vi "kreator_siatki.vi"(2 "error in (no error)":errorcluster, 3 "Liczba Przejść":i32, 4 "Wektor 2":dbl[](array[numeric]), 5 "Wektor 1":dbl[](array[numeric])) -> (0 "error out":errorcluster, 1 "Tablica pkt":dbl[][][](array[numeric]))   [LabVIEW 2016]
doc: "To subvi zwraca tablice pkt. stworzonych z przyjętych wektorów bazowych , oddalonych od zera od zadanej liczbie przejść"
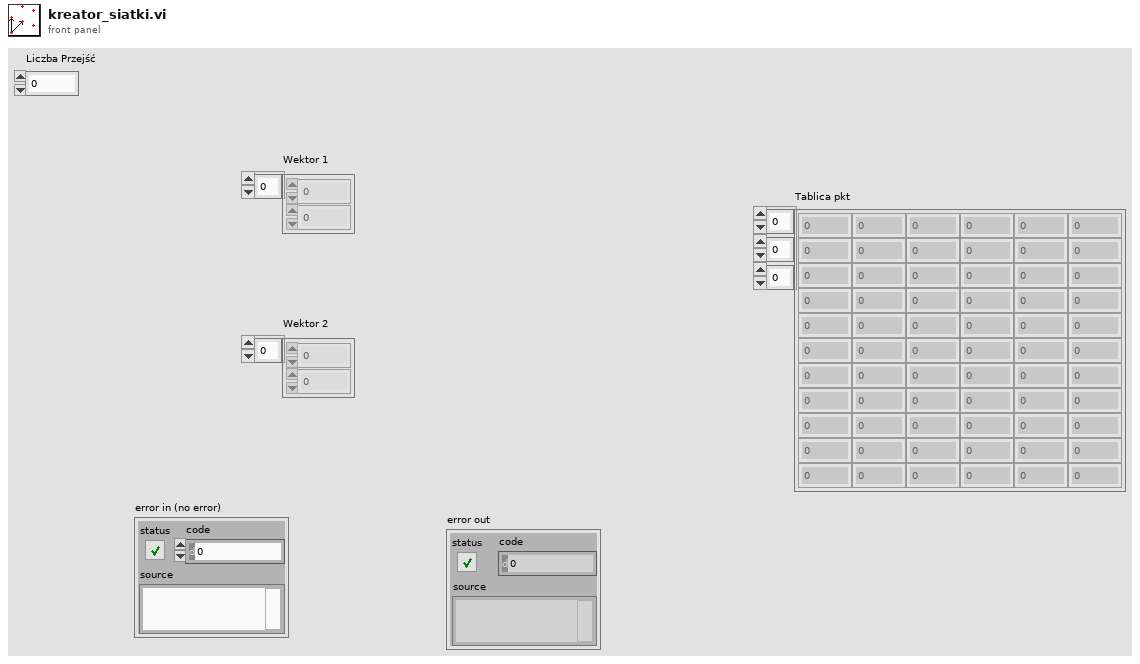
[diagram p1: front panel]
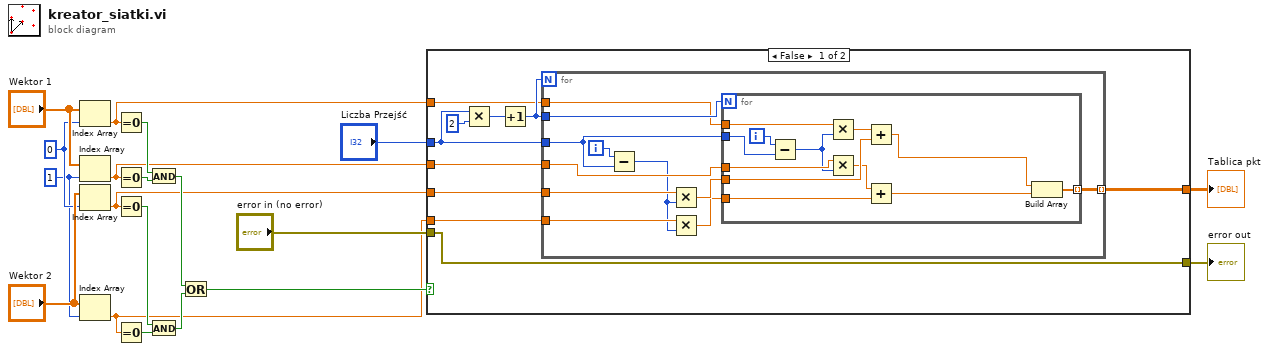
[diagram p0: block diagram]
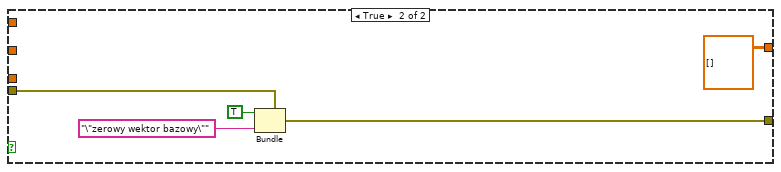
[diagram p2: hidden frame]
diagram:
  w16 = 1 ("index")
  w17 = 0 ("index")
  n1 = Index Array(array="Wektor 1", index=w17) -> (element=w5:dbl)
  n2 = Index Array(array="Wektor 1", index=w16) -> (element=w4:dbl)
  n3 = Index Array(array="Wektor 2", index=w17) -> (element=w3:dbl)
  n4 = Index Array(array="Wektor 2", index=w16) -> (element=w2:dbl)
  n5 = Equal To 0?(x=w5) -> (x = 0?=w15:bool)
  n6 = Equal To 0?(x=w4) -> (x = 0?=w14:bool)
  n7 = Equal To 0?(x=w3) -> (x = 0?=w13:bool)
  n8 = Equal To 0?(x=w2) -> (x = 0?=w12:bool)
  n9 = And(x=w15, y=w14) -> (x .and. y?=w11:bool)
  n10 = And(x=w13, y=w12) -> (x .and. y?=w10:bool)
  n11 = Or(x=w11, y=w10) -> (x .or. y?=w9:bool)
  n12 = case shown="False" w9 {
    tunnel: "error in (no error)" -> [w29 w57]
    tunnel: [w29 w54] -> w7
    tunnel: "Liczba Przejść" -> [w20 _]
    tunnel: w5 -> [w27 _]
    tunnel: w4 -> [w26 _]
    tunnel: w3 -> [w25 _]
    tunnel: w2 -> [w24 _]
    tunnel: [w23 dbl[][][] []] -> w1
    frame False {
      n13 = Multiply(x=w20, y=2) -> (x*y=w21:i32)
      n14 = Increment(x=w21) -> (x+1=w28:i32)
      n15 = for {
        N: w28 -> [_]
        tunnel: w28 -> [w40]
        tunnel: w27 -> [w39]
        tunnel: w26 -> [w38]
        tunnel: w25 -> [w37]
        tunnel: w24 -> [w36]
        tunnel: [w33] -> w23 mode=indexing
        tunnel: w20 -> [w32]
        i -> [w31]
        n16 = Subtract(x=w31, y=w32) -> (x-y=w30:i32)
        n17 = Multiply(x=w37, y=w30) -> (x*y=w35:dbl)
        n18 = Multiply(x=w36, y=w30) -> (x*y=w34:dbl)
        n19 = for {
          N: w40 -> [_]
          tunnel: w39 -> [w52]
          tunnel: w38 -> [w51]
          tunnel: w35 -> [w49]
          tunnel: w34 -> [w48]
          tunnel: [w44] -> w33 mode=indexing
          tunnel: w32 -> [w43]
          i -> [w42]
          n20 = Subtract(x=w42, y=w43) -> (x-y=w41:i32)
          n21 = Multiply(x=w52, y=w41) -> (x*y=w50:dbl)
          n22 = Multiply(x=w51, y=w41) -> (x*y=w47:dbl)
          n23 = Add(x=w50, y=w49) -> (x+y=w46:dbl)
          n24 = Add(x=w47, y=w48) -> (x+y=w45:dbl)
          n25 = Build Array(w46, w45) -> (w44:dbl[])
        }
      }
    }
    frame True {
      n26 = Bundle(cluster=w57, "status"=TRUE, "source"="\"zerowy wektor bazowy\"") -> (w54:errorcluster)  [unwired: 1 in]
    }
  }
  "error out" <- w7
  "Tablica pkt" <- w1
